vi "process_image.vi"(0 "Image Data In":T4, 7 "Image Processing Data In":T2, 11 "Threshold range":cluster{"Lower value":sgl, "Upper value":sgl}={"Lower value"=6.0, "Upper value"=1024.0}) -> (4 "Image Data Out":T4, 8 "Image Processing Data Out":T2, 12 "Accumulated Image Out":i16[][](array[numeric]), 13 "Particle Measurements (Pixels)":dbl[][](array[numeric]), 14 "Number of Particles":u16, 15 "Output data":T1)   [LabVIEW 2023]
uses:
  <vilib>/vision/Image Controls.llb/IMAQ Image.ctl
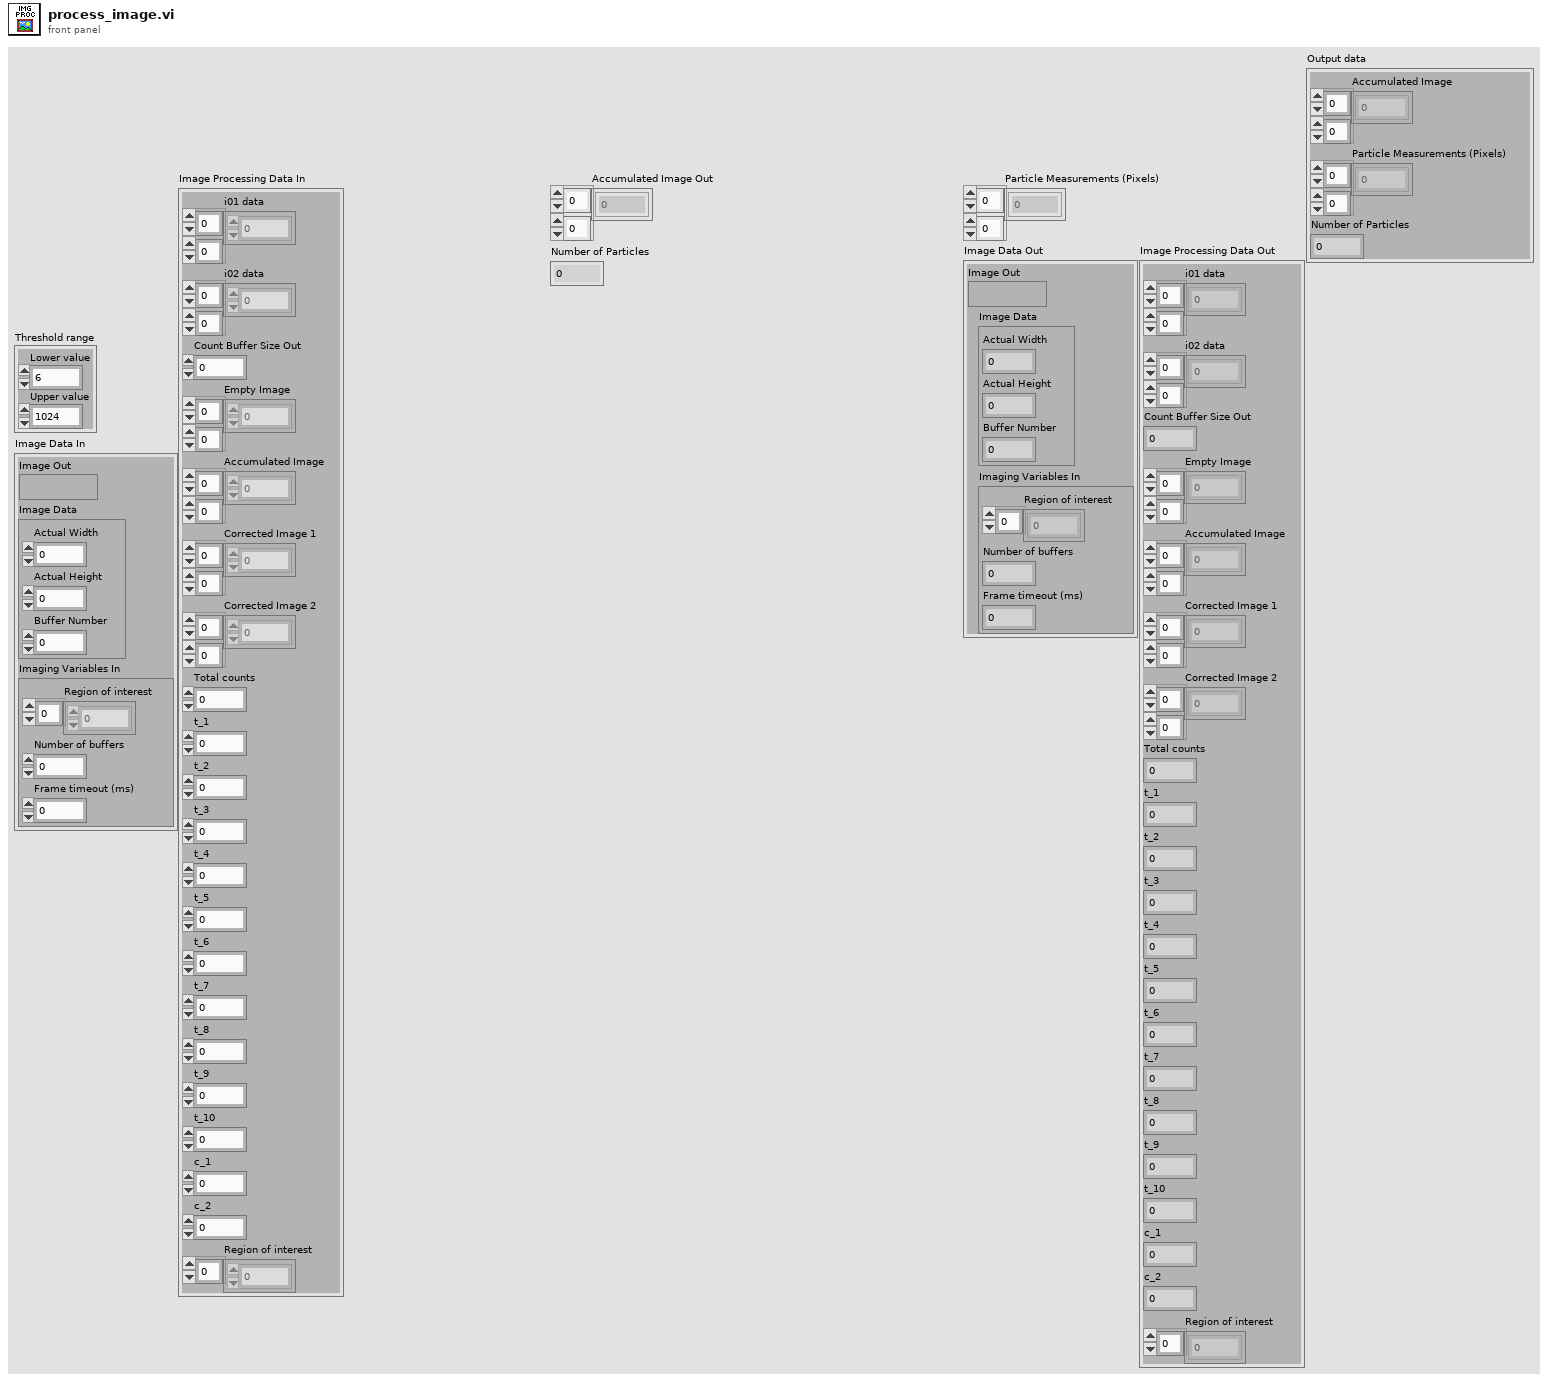
[diagram p1: front panel]
types:
  T1 = cluster{"Accumulated Image":i16[][], "Particle Measurements (Pixels)":dbl[][], "Number of Particles":u16}
  T2 = cluster{"i01 data":sgl[][], "i02 data":sgl[][], "Count Buffer Size Out":i32, "Empty Image":i16[][], "Accumulated Image":i16[][], "Corrected Image 1":i16[][], "Corrected Image 2":i16[][], "Total counts":i32, "t_1":i32, "t_2":i32, "t_3":i32, "t_4":i32, "t_5":i32, "t_6":i32, "t_7":i32, "t_8":i32, "t_9":i32, "t_10":i32, "c_1":i32, "c_2":i32, "Region of interest":i32[]}
  T3 = typedef "IMAQ Image.ctl" = refnum<image>
  T4 = cluster{"Image Out":T3, "Image Data":cluster{"Actual Width":u32, "Actual Height":u32, "Buffer Number":i32}, "Imaging Variables In":cluster{"Region of interest":i32[], "Number of buffers":u32, "Frame timeout (ms)":u32}}
  T5 = cluster{"Region of interest":i32[], "Number of buffers":u32, "Frame timeout (ms)":u32}
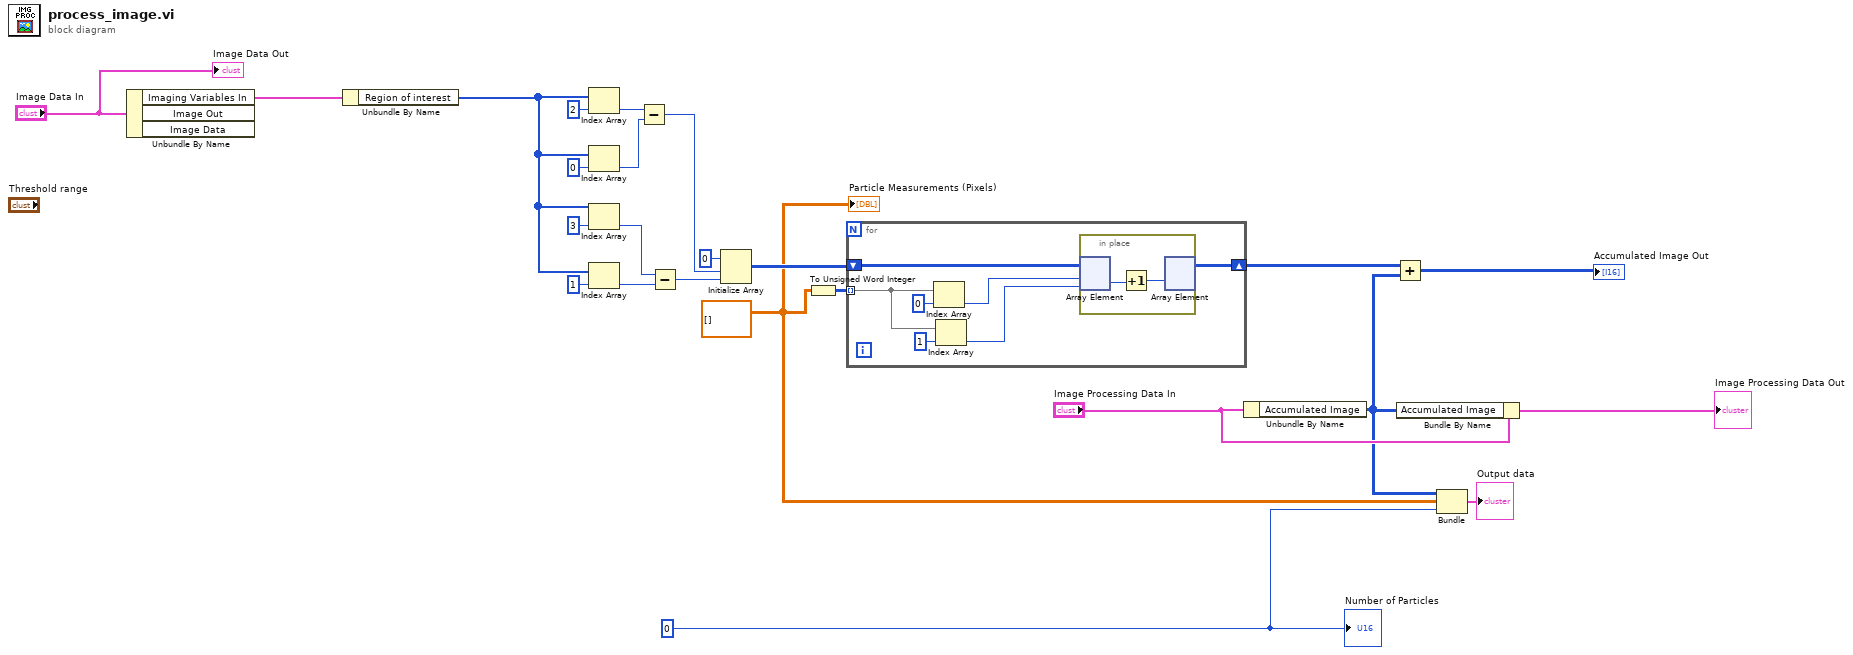
[diagram p0: block diagram]
diagram:
  w2 = u16 0 ("Number of Particles")
  w3 = dbl[][] [] ("Particle Measurements (Pixels)")
  n1 = Unbundle By Name("Image Data In") -> ("Imaging Variables In"=w9:T5)  [unwired: 2 out]
  n2 = Unbundle By Name(w9) -> ("Region of interest"=w13:i32[])
  n3 = Index Array(array=w13, index=2) -> (element=w20:i32)
  n4 = Index Array(array=w13, index=0) -> (element=w19:i32)
  n5 = Index Array(array=w13, index=3) -> (element=w17:i32)
  n6 = Index Array(array=w13, index=1) -> (element=w18:i32)
  n7 = Subtract(x=w20, y=w19) -> (x-y=w15:i32)
  n8 = Subtract(x=w17, y=w18) -> (x-y=w14:i32)
  n9 = Initialize Array(i16 0 ("element"), w15, w14) -> (w12:i16[][])
  n10 = To Unsigned Word Integer(number=w3) -> (unsigned 16bit integer=w11:u16[][])
  n11 = for {
    tunnel: w11 -> [w30] mode=indexing
    shift-right: [w27] -> w7
    shift-left: w12 -> [w28]
    n12 = Index Array(array=w30, index=0) -> (element=w26:u16)
    n13 = Index Array(array=w30, index=1) -> (element=w25:u16)
    n14 = in-place {
      n15 = in-place-array #1(w28, w26, w25) -> (w33:i16)
      n16 = Increment(x=w33) -> (x+1=w32:i16)
      n17 = in-place-array #1(w32) -> (w27:i16[][])  [unwired: 2 out]
    }
  }
  n18 = Unbundle By Name("Image Processing Data In") -> ("Accumulated Image"=w4:i16[][])
  n19 = Add(x=w7, y=w4) -> (x+y=→"Accumulated Image Out":i16[][])
  n20 = Bundle By Name(cluster="Image Processing Data In", "Accumulated Image"=w4) -> (→"Image Processing Data Out":T2)
  n21 = Bundle("Accumulated Image"=w4, "Particle Measurements (Pixels)"=w3, "Number of Particles"=w2) -> (→"Output data":T1)  [unwired: 1 in]
  "Number of Particles" <- w2
  "Particle Measurements (Pixels)" <- w3
  "Image Data Out" <- "Image Data In"
